vi "TRABALHO AULA 2 ARTHUR.vi"() -> ()   [LabVIEW 2025]
panel:
  in  "Boolean":bool
  in  "Numeric":dbl
  in  "stop 3":bool
  out "Numeric 3":i32
  out "ºC 3":dbl(slide) scale=0.0..100.0
  in  "ºF 3":dbl(slide) scale=0.0..110.0
  out "x*y 3":dbl
  in  "stop 2":bool
  out "Numeric 2":i32
  out "ºC 2":dbl(slide) scale=0.0..100.0
  in  "ºF 2":dbl(slide) scale=0.0..110.0
  out "x*y 2":dbl
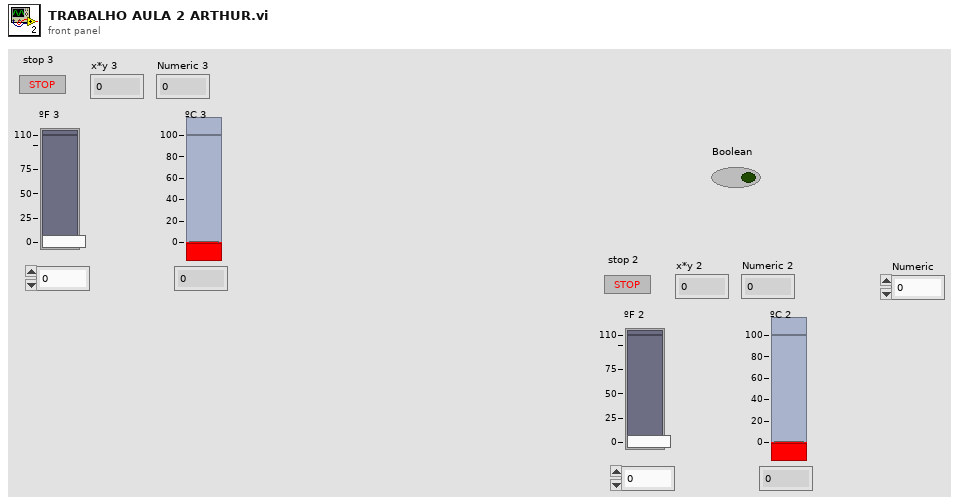
[diagram p1: front panel]
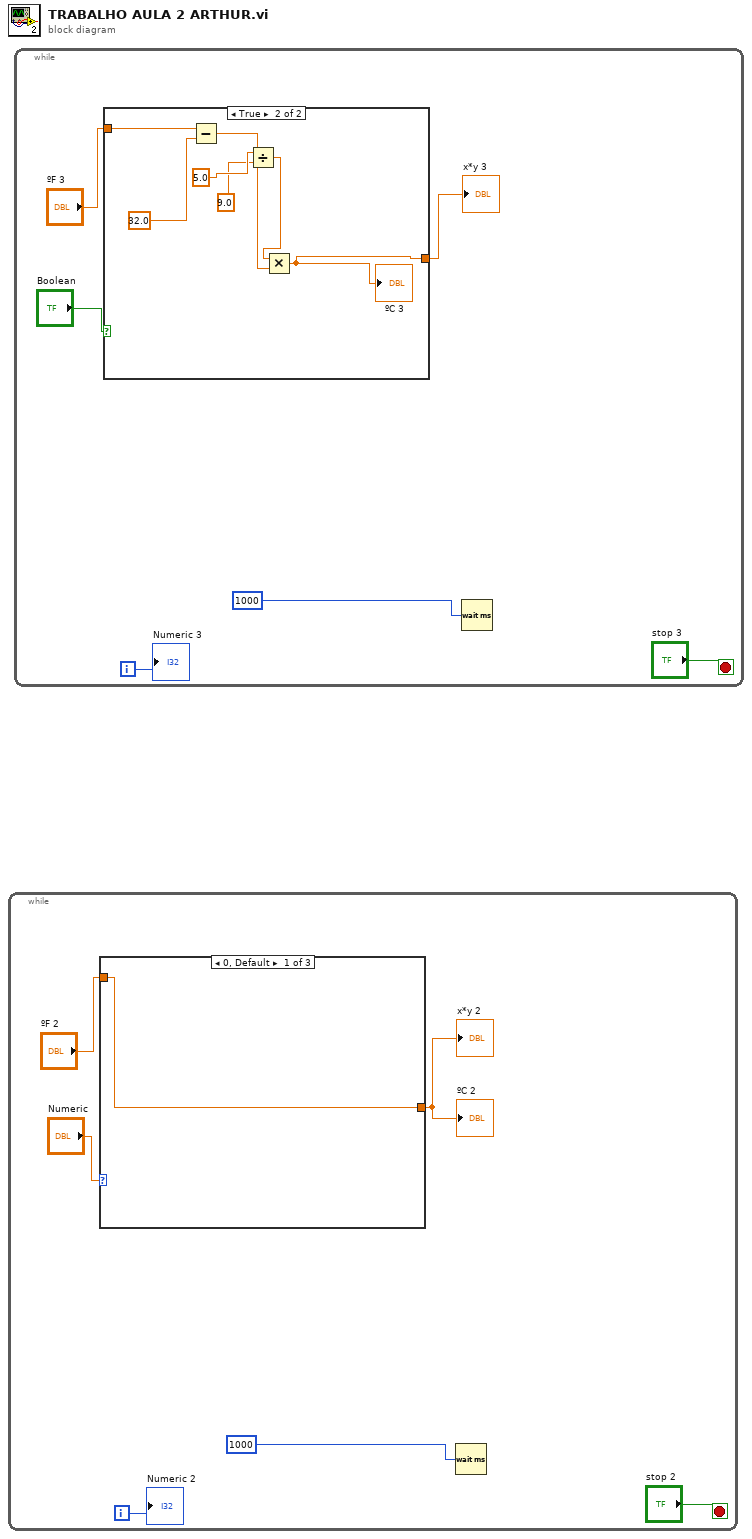
[diagram p0: block diagram]
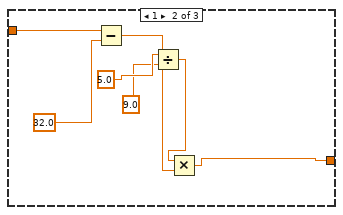
[diagram p3: hidden frame]
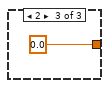
[diagram p4: hidden frame]
diagram:
  n1 = while {
    i -> [w5]
    stop <- "stop 2" stop-if-true
    n2 = case shown="0, Default" "Numeric" {
      tunnel: "ºF 2" -> [w7 w9 _]
      tunnel: [w7 w8 0.0 ("ºF 2")] -> w2
      frame 0, Default {
      }
      frame 1 {
        n3 = Subtract(x=w9, y=32.0) -> (x-y=w11:dbl)
        n4 = Divide(x=5.0, y=9.0) -> (x/y=w12:dbl)
        n5 = Multiply(x=w12, y=w11) -> (x*y=w8:dbl)
      }
      frame 2 {
      }
    }
    "x*y 2" <- w2
    "ºC 2" <- w2
    n6 = Wait (ms)(milliseconds to wait=u32 1000) -> ()  [unwired: 1 out]
    "Numeric 2" <- w5
  }
  n7 = while {
    i -> [w20]
    stop <- "stop 3" stop-if-true
    n8 = case shown="True" "Boolean" {
      tunnel: "ºF 3" -> [w22 w24]
      tunnel: [w22 w23] -> w17
      frame False {
      }
      frame True {
        n9 = Subtract(x=w24, y=32.0) -> (x-y=w26:dbl)
        n10 = Divide(x=5.0, y=9.0) -> (x/y=w27:dbl)
        n11 = Multiply(x=w27, y=w26) -> (x*y=w23:dbl)
        "ºC 3" <- w23
      }
    }
    "x*y 3" <- w17
    n12 = Wait (ms)(milliseconds to wait=u32 1000) -> ()  [unwired: 1 out]
    "Numeric 3" <- w20
  }
